vi "Dashboard Main.vi"() -> ()   [LabVIEW 2016]
uses:
  <vilib>/Utility/miscctls.llb/LVRowAndColumnTypeDef.ctl
  <vilib>/event_ctls.llb/eventvkey.ctl
  <vilib>/Rock Robotics/Network Tables/NT Read Boolean.vi
  <vilib>/Rock Robotics/Network Tables/NT Write Boolean.vi
  <vilib>/Rock Robotics/Network Tables/NT Read Numeric Array.vi
  <vilib>/Rock Robotics/WPI/Dashboard/WPI_DashboardLogging Global.vi
panel:
  in  "Camera Settings Right":T1={"Frame Rate"=30, "Compression"=30, "Size"=1, "DB Camera Config"=FALSE} {"Frame Rate" scale=1.0..30.0; "Compression" scale=100.0..-1.0; "Size" items=["640x480", "320x240", "160x120"]}
  in  "Camera Name Right":string(combo)="No Camera Selection"
  out "Camera Info":cluster{"Mbps LED":bool, "Mbps":dbl, "fps":dbl} {"fps" format="%#.1g"; "Mbps" format="%#.1g"}
  in  "Camera Settings":T1={"Frame Rate"=30, "Compression"=30, "Size"=1, "DB Camera Config"=FALSE} {"Frame Rate" scale=1.0..30.0; "Compression" scale=100.0..-1.0; "Size" items=["640x480", "320x240", "160x120"]}
  in  "TCP":refnum<k5>
  in  "Rec Mode":enum32{"Stop", "Record", "Playback"}(radio)
  out "Robot IP":string
  out "Image Message":string="Timeout in Camera Communications"
  in  "Dashboard Tab":T2(tab)
  in  "Select Auto":string(combo)="Select Autonomous ..."
  out "NT Connection":bool
  out "MotorChart R":cluster{"Numeric":dbl, "Numeric":dbl}(graph)
  out "MotorChart L":cluster{"Numeric":dbl, "Numeric":dbl}(graph)
  out "MotorSliders R":cluster{"MotorSlide1":dbl, "MotorSlide2":dbl} {"MotorSlide2" scale=-1.0..1.0 scale format="%#_2e"; "MotorSlide1" scale=-1.0..1.0 scale format="%#_2e"}
  out "MotorSliders L":cluster{"MotorSlide1":dbl, "MotorSlide2":dbl} {"MotorSlide2" scale=-1.0..1.0 scale format="%#_2e"; "MotorSlide1" scale=-1.0..1.0 scale format="%#_2e"}
  out "Gyro":dbl(knob) scale=0.0..360.0
  out "JS1 Z":dbl(slide) scale=-1.0..1.0 scale format="%#_2e"
  out "JS1 Graph":cluster{"X":dbl, "Y":dbl}[](graph)
  out "JS1 Buttons":T3
  out "JS2 Z":dbl(slide) scale=-1.0..1.0 scale format="%#_2e"
  out "JS2 Graph":cluster{"X":dbl, "Y":dbl}[](graph)
  out "JS2 Buttons":T3
  out "Mode":T4(ring)=enum."Auto Disabled"
  out "Camera Image Right":T5(plugin-control)
  in  "DB/String 9":string
  in  "DB/String 8":string
  in  "DB/String 7":string
  in  "DB/String 6":string
  in  "DB/String 5":string
  in  "DB/String 4":string
  in  "DB/String 3":string
  in  "DB/String 2":string
  in  "DB/String 1":string
  in  "DB/String 0":string
  in  "DB/Slider 0":dbl(slide) scale=0.0..5.0
  in  "DB/Slider 1":dbl(slide) scale=0.0..5.0
  in  "DB/Slider 2":dbl(slide) scale=0.0..5.0
  in  "DB/Slider 3":dbl(slide) scale=0.0..5.0
  out "DB/LED 3":bool
  out "DB/LED 2":bool
  out "DB/LED 1":bool
  out "DB/LED 0":bool
  in  "DB/Button 3":bool
  in  "DB/Button 2":bool
  in  "DB/Button 1":bool
  in  "DB/Button 0":bool caption="New Name"
  in  "Capture":bool=TRUE
  in  "Test Slider":dbl(slide) scale=0.0..100.0 scale format="%#_3g"
  in  "On/Off":bool caption="Solenoid"
  in  "Test Name":u16(ring) items=["Select the test to run..."]
  in  "Test Tree":string(tree)
  in  "Motor":cluster{"Value":dbl, "Enable":bool} {"Value" scale=-1.0..1.0 scale format="%#_3g"}
  out "Progress":T6 {"Test Progress" scale=0.0..100.0}
  in  "Rev/Fwd":cluster{"Forward":bool, "Reverse":bool}
  in  "Test Ring":u16(ring) items=["Monochrome", "Color"]
  out "Cmd Status":string
  in  "Execute Command":bool
  in  "Command Params":string[][](table)
  in  "Command Selection":i32(listbox)
  in  "CheckList":i32(listbox)
  out "Tree":string(tree)
  out "Camera Image":T5(plugin-control)
  out "Background":bool
  in  "Camera Name":string(combo)="No Camera Selection"
  # "HW"
  # "HW"
  # "Joysticks"
  # "Drive Motors"
  # "Front"
  # "Right"
  # "Left"
  # "Back"
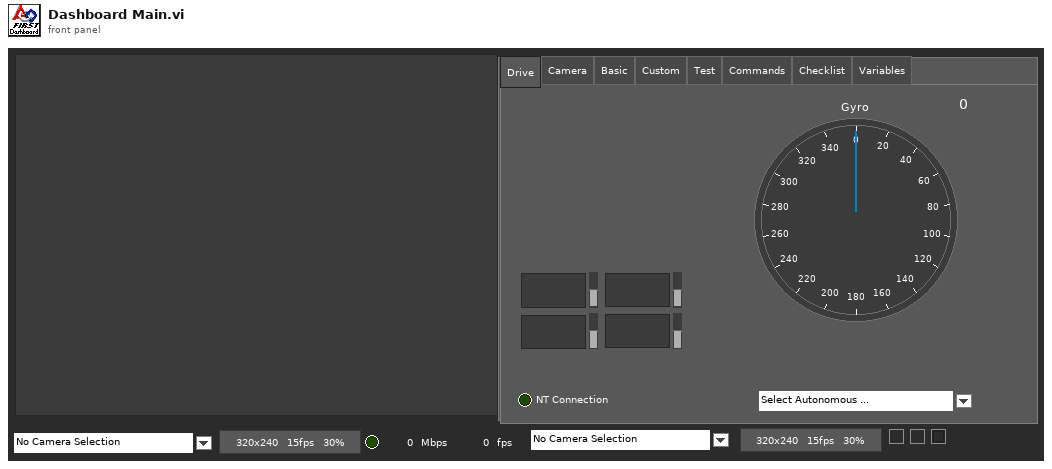
[diagram p1: front panel]
types:
  T1 = cluster{"Frame Rate":i32, "Compression":i32, "Size":u16, "DB Camera Config":bool}
  T2 = enum32{"Drive", "Camera", "Basic", "Custom", "Test", "Commands", "Checklist", "Variables"}
  T3 = cluster{bool, bool, bool, bool, bool, bool, bool, bool, bool, bool, bool, bool}
  T4 = enum8{"Tele-Op Disabled", "Tele-Op Enabled", "Auto Disabled", "Auto Enabled", "Test Disabled", "Test Enabled", "Disconnected", "No Code", "E-Stop"}
  T5 = typedef "IMAQ Image.ctl" = refnum<image>
  T6 = cluster{"Test Progress":u8, "Test Progress Text":string}
  T7 = typedef "Image Type" = u32
  T8 = cluster{"IDs":cluster{"RPC field ID":u16, "Unique ID":u16}, "String":string}
  T9 = enum32{"Drive", "Basic", "Custom", "Test", "Checklist", "Variables"}
  T10 = enum16{"open", "replace", "create", "open or create", "replace or create", "replace or create with confirmation"}
  T11 = cluster{"Error Strings":string, "Disable Counts":cluster{u16, u16}, "Rail Faults":cluster{u16, u16, u16}, "Robot IP":string, "DB Mode":u8, "Event Info":cluster{"Name":string, "Type":u8, "Number":u16, "Replay":u8}}
  T12 = cluster{"Storage":cluster{"Disk Free":u64, "RAM Block":u32, "RAM free":u32}, "CPU Utilization":cluster{"CPU % ISR":sgl, "CPU % Time Crit":sgl, "CPU % Timed Str":sgl, "CPU % High":sgl, "CPU % Above":sgl, "CPU % Normal":sgl, "CPU % Low":sgl}, "CAN":cluster{"% Bus Utilization":sgl, "Bus Off Cnt":u32, "TX_FIFO Full Cnt":u32, "Receive Error Cnt":u8, "Transmit Error Cnt":u8}, "HID":cluster{"HID Outputs":u32, "Rumble Low":u16, "Rumble High":u16}[]}
  T13 = cluster{"Status bits":cluster{"Test Mode":bool, "Autonomous":bool, "Enabled":bool, "Code Start":bool, "Brownout":bool, "Reserved 2":bool, "Reserved 3":bool, "E-Stop":bool}, "Code Trace":cluster{"Disabled":bool, "TeleOp":bool, "Auto":bool, "Test":bool}, "Controller Type":enum16{"unknown", "cRIO", "roboRio"}, "Code?":enum16{"unknown", "noCode", "code"}, "Battery V":dbl}
  T14 = cluster{"Control Bits":cluster{"TestMode":bool, "Autonomous":bool, "Enabled":bool, "FMS Present":bool, bool, bool, bool, "E-Stop":bool}, "Team Station ":u8, "Countdown":sgl, "Joystick Values":cluster{"Axes":dbl[], "Buttons":bool[], "POVs":i16[]}[]}
  T15 = cluster{"Axes":dbl[], "Buttons":bool[], "POVs":i16[]}[]
  T16 = cluster{"Axes":dbl[], "Buttons":bool[], "POVs":i16[]}
  T17 = cluster{"Buttons[0]":bool, "Buttons[1]":bool, "Buttons[2]":bool, "Buttons[3]":bool, "Buttons[4]":bool, "Buttons[5]":bool, "Buttons[6]":bool, "Buttons[7]":bool, "Buttons[8]":bool, "Buttons[9]":bool, "Buttons[10]":bool, "Buttons[11]":bool}
  T18 = cluster{"Camera Image":refnum<vi>, "Dashboard Tab":refnum<vi>, "Background":refnum<vi>, "Rec Mode":refnum<vi>, "Test Slider":refnum<vi>, "On/Off ":refnum<vi>, "Test Ring":refnum<vi>, "Rev/Fwd":refnum<vi>, "Test Name":refnum<vi>, "Motor":refnum<vi>, "Progress":refnum<vi>, "CheckList":refnum<vi>, "Tree":refnum<vi>, "Test Tree":refnum<vi>, "Command Params":refnum<vi>, "Command Selection":refnum<vi>, "Execute Command":refnum<vi>, "Cmd Status":refnum<vi>, "Camera Settings":refnum<vi>, "Camera Name":refnum<vi>, "Camera Info":refnum<vi>, "Camera Settings Right":refnum<vi>, "Camera Name Right":refnum<vi>, "Camera Image Right":refnum<vi>}
  T19 = cluster{"Operation":enum16{"Update", "Clear"}, "Color Box":u32}[]
  T20 = typedef "eventvkey.ctl" = enum16{"ASCII", "Enter", "Return", "Shift", "Ctrl", "Alt", "Cmd", "Opt", "Caps", "NumLock", "Clear", "Break", "Up", "Down", "Left", "Right", "Insert", "Delete", "Home", "End", "PageUp", "PageDown", "Escape", "Help", "Pause", "ScrollLock", "F1", "F2", "F3", "F4", "F5", "F6", "F7", "F8", "F9", "F10", "F11", "F12", "F13", "F14", "F15", "F16", "F17", "F18", "F19", "F20", "F21", "F22", "F23", "F24", "Play", "VolumeUp", "VolumeDown", "Mute", "Two Byte Char"}
  T21 = cluster{"Image Size":bool, "Image Type":bool, "Pixel Value":bool, "ROI Information":bool, "Zoom Factor":bool}
  T22 = cluster{"Operation":enum16{"Update", "Clear"}, "Color Box":u32}
  T23 = typedef "LVRowAndColumnTypeDef.ctl" = cluster{"Row":i32, "Column":i32}
  T24 = cluster{"Shift":bool, "Ctrl":bool, "Alt":bool, "Cmd":bool, "Opt":bool}
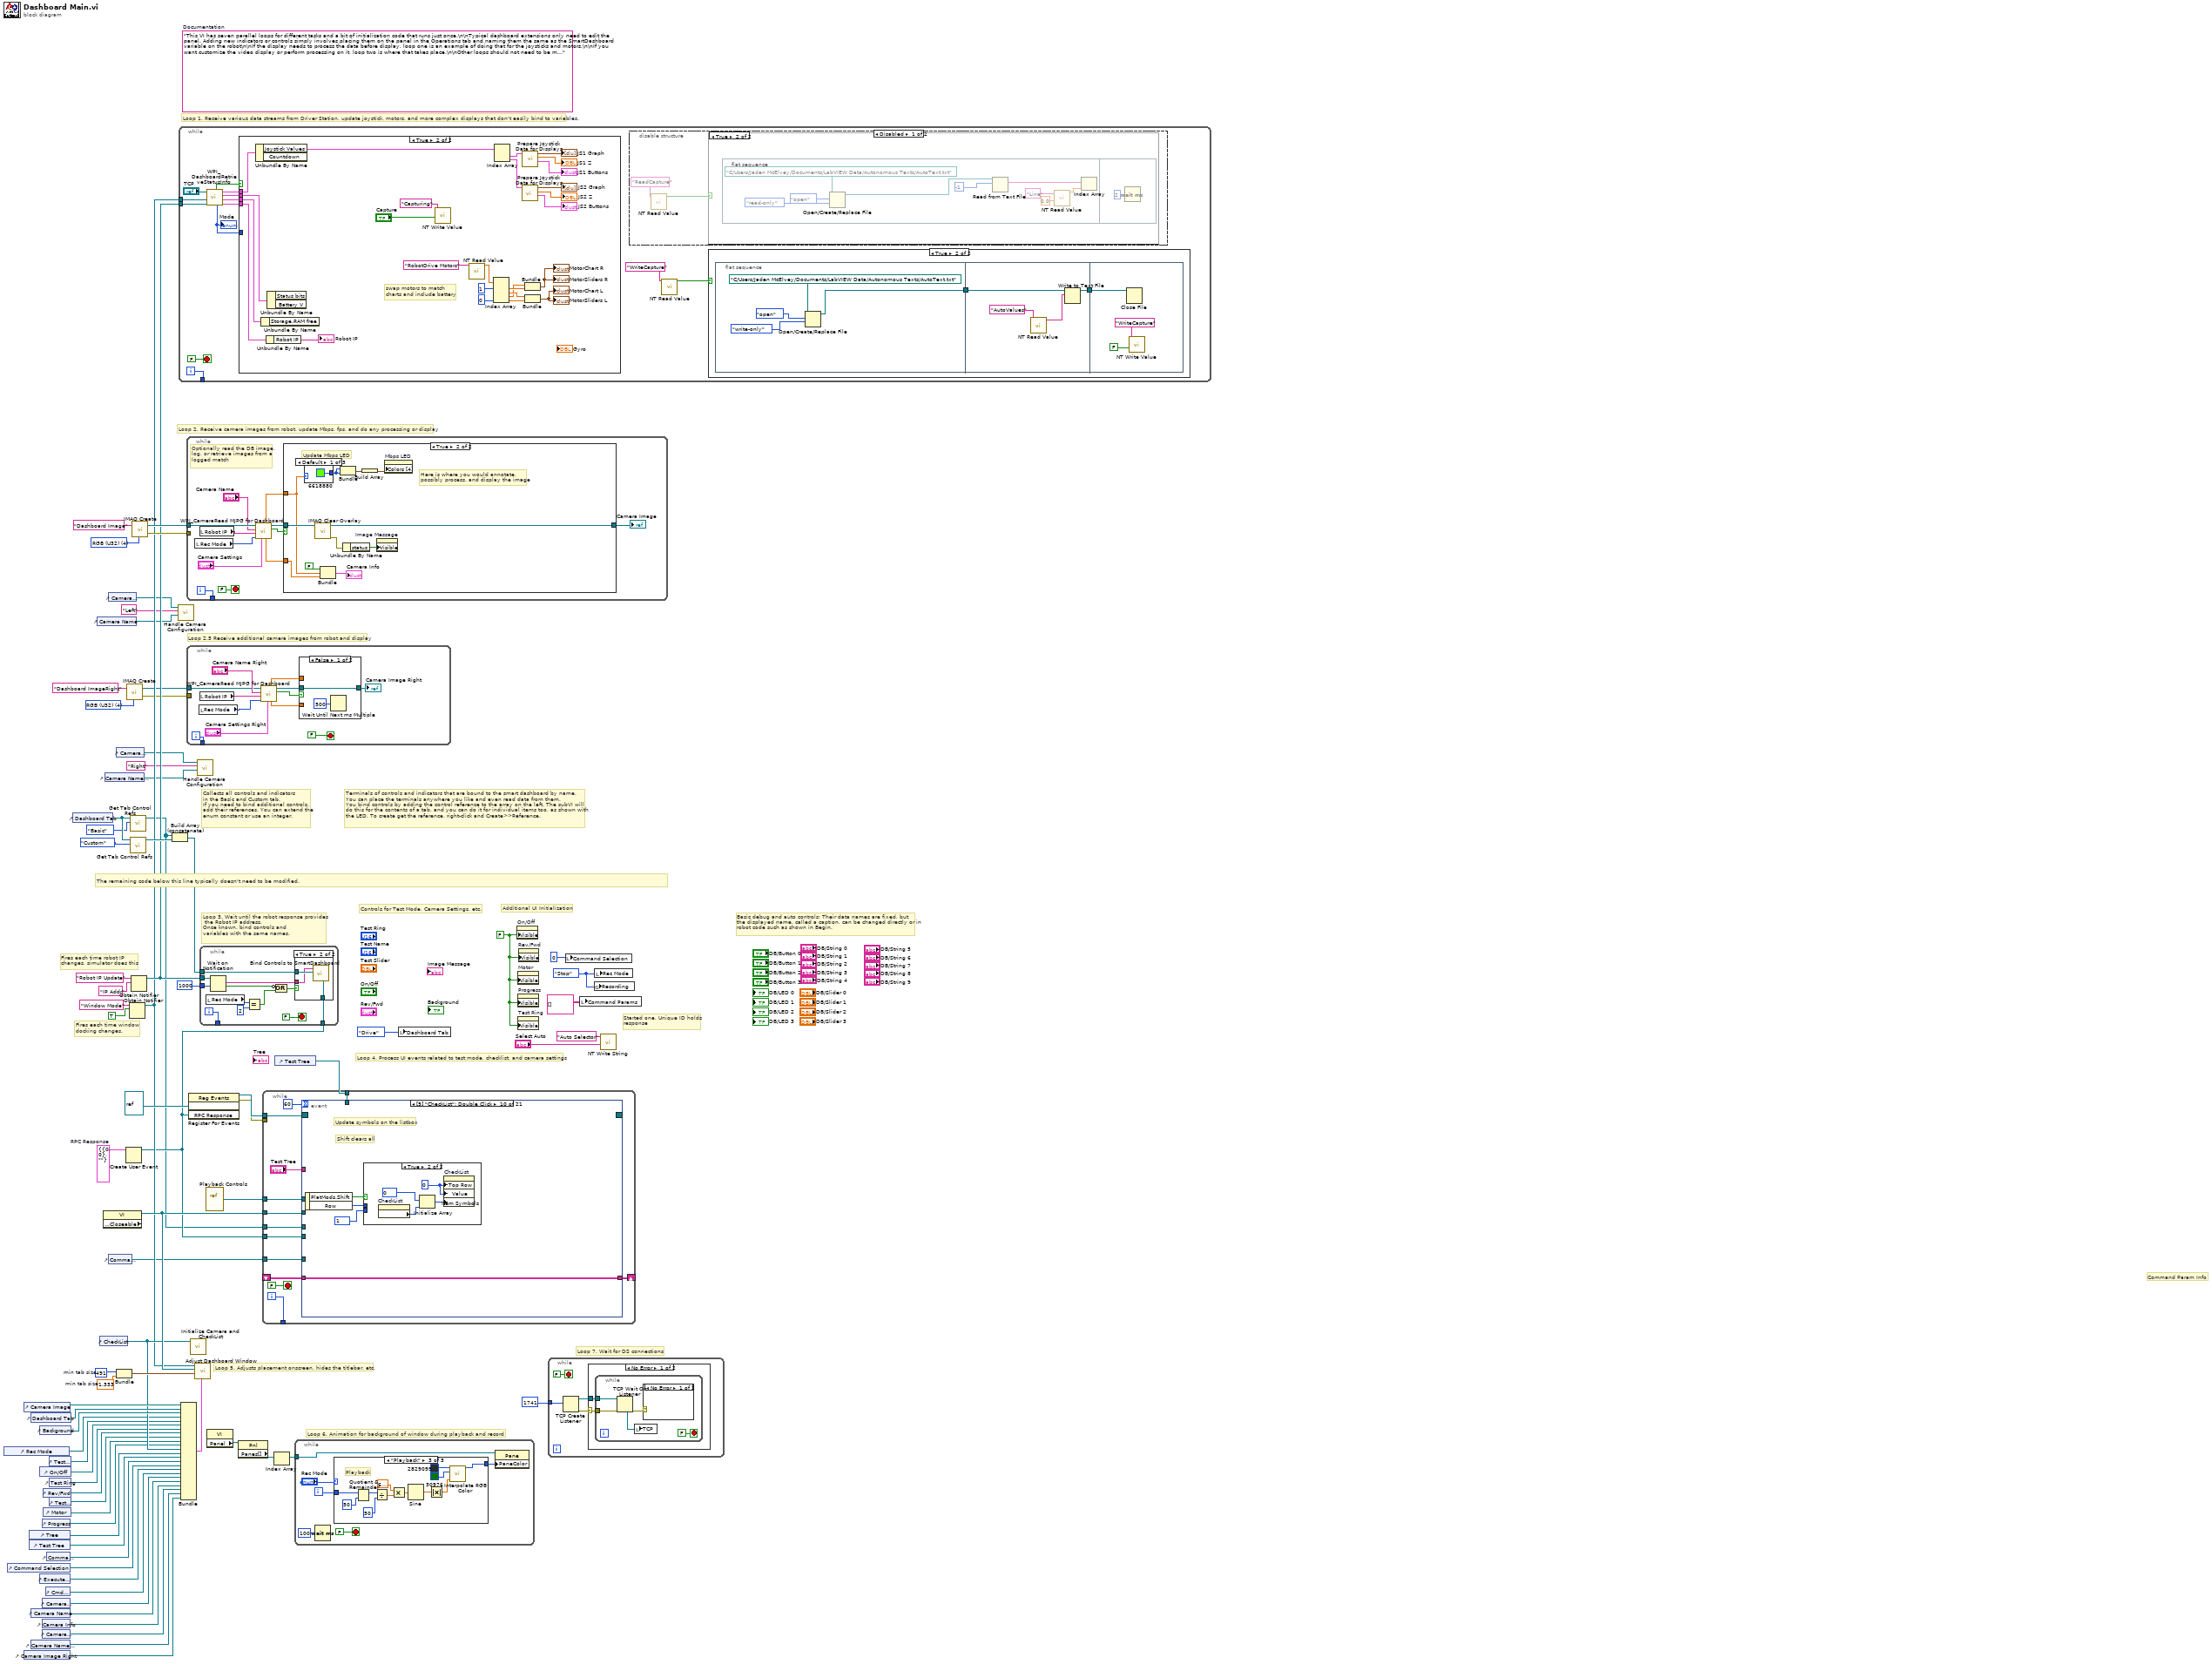
[diagram p0: block diagram]
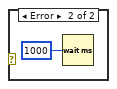
[diagram p3: hidden frame]
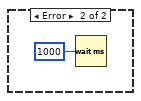
[diagram p4: hidden frame]
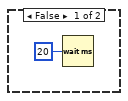
[diagram p8: hidden frame]
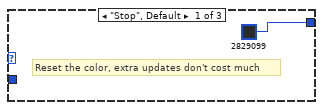
[diagram p9: hidden frame]
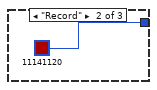
[diagram p10: hidden frame]
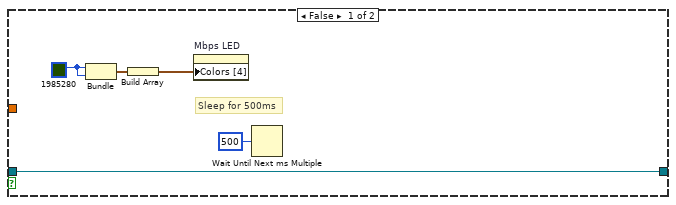
[diagram p12: hidden frame]
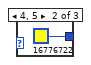
[diagram p13: hidden frame]
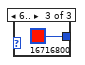
[diagram p14: hidden frame]
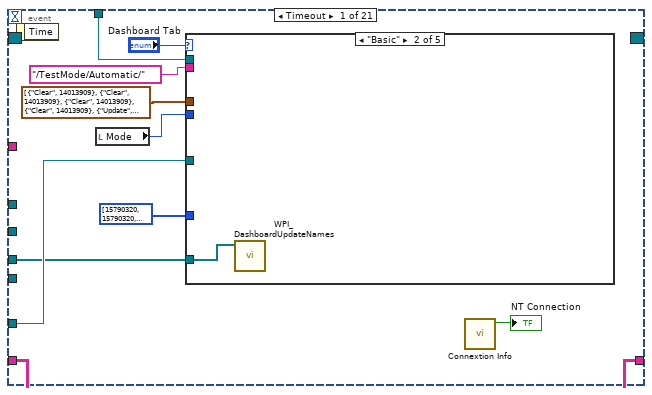
[diagram p15: hidden frame]
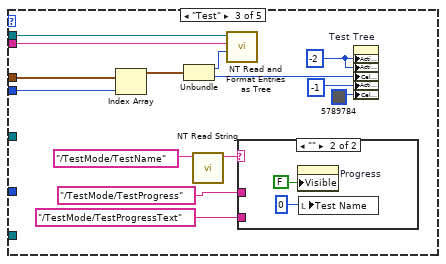
[diagram p17: hidden frame]
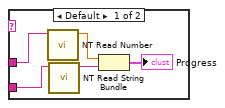
[diagram p18: hidden frame]
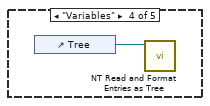
[diagram p19: hidden frame]
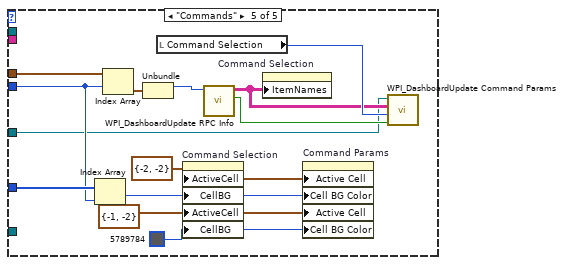
[diagram p20: hidden frame]
diagram:
  w11 = T7 4 items=["Grayscale (U8)", "Grayscale (I16)", "Grayscale (SGL)", "Complex (CSG)", "RGB (U32)", "HSL (U32)", "RGB (U64)"] ("Image Type")
  w26 = T8 {"IDs"={"RPC field ID"=0, "Unique ID"=0}, "String"=""}  # RPC Response
  w51 = 491  # min tab size
  w50 = 1.333  # min tab size
  w58 = enum32{"Stop", "Record", "Playback"}."Stop" ("Rec Mode")
  w33 = FALSE ("Visible")
  (unwired) "This VI has seven parallel loops for different tasks and a bit of initialization code that runs just once.\n\nTypical dashboard extensions only need to edit the panel. Adding new indicators or controls simply involves placing them on the panel in the Operations tab and naming them the same as the SmartDashboard variable on the robot\n\nIf the display needs to process the data before display, loop one is an example of doing that for the joysticks and motors.\n\nIf you want customize the video display or perform processing on it, loop two is where that takes place.\n\nOther loops should not need to be modified. They are pretty standard, and document the task they perform."  # Documentation
  w75 = T7 4 items=["Grayscale (U8)", "Grayscale (I16)", "Grayscale (SGL)", "Complex (CSG)", "RGB (U32)", "HSL (U32)", "RGB (U64)"] ("Image Type")
  # "Loop 2.5 Receive additional camera images from robot and display"
  # "Command Param Info"
  # "Started one, Unique ID holds\nresponse"
  # "Loop 7. Wait for DS connections"
  # "Basic debug and auto controls: Their data names are fixed, but\nthe displayed name, called a caption, can be changed directly or in\nrobot code such as shown in Begin."
  # "Controls for Test Mode, Camera Settings, etc."
  # "Additional UI Initialization"
  # "Loop 6. Animation for background of window during playback and record"
  # "Fires each time robot IP\nchanges, simulator does this"
  # "Fires each time window\ndocking changes."
  # "Collects all controls and indicators\nin the Basic and Custom tab.\nIf you need to bind additional controls,\nadd their references. You can extend the\nenum constant or use an integer."
  # "The remaining code below this line typically doesn't need to be modified."
  # "Loop 4. Process UI events related to test mode, checklist, and camera settings"
  # "Terminals of controls and indicators that are bound to the smart dashboard by name.\nYou can place the terminals anywhere you like and even read data from them.\nYou bind controls by adding the control reference to the array on the left. The subVI will\ndo this for the contents of a tab, and you can do it for individual items too, as shown with\nthe LED. To create get the reference, right-click and Create>>Reference."
  # "Loop 3. Wait until the robot response provides\n the Robot IP address.\nOnce known, bind controls and\nvariables with the same names."
  # "Loop 5. Adjusts placement onscreen, hides the titlebar, etc."
  # "Loop 1. Receive various data streams from Driver Station, update joystick, motors, and more complex displays that don't easily bind to variables."
  # "Loop 2. Receive camera images from robot, update Mbps, fps, and do any processing or display"
  n1 = control-ref of="Rec Mode"() -> (w39:refnum<vi>)
  n2 = control-ref of="Command Selection"() -> (w25:refnum<vi>)
  n3 = control-ref of="Camera Image Right"() -> (w2:refnum<vi>)
  n4 = control-ref of="Camera Image"() -> (w53:refnum<vi>)
  n5 = control-ref of="Tree"() -> (w43:refnum<vi>)
  n6 = control-ref of="Test Tree"() -> (w42:refnum<vi>)
  n7 = control-ref of="Dashboard Tab"() -> (w52:refnum<vi>)
  n8 = control-ref of="Camera Name"() -> (w16:refnum<vi>)
  n9 = control-ref of="Camera Name Right"() -> (w3:refnum<vi>)
  n10 = control-ref of="Execute Command"() -> (w27:refnum<vi>)
  n11 = control-ref of="Background"() -> (w48:refnum<vi>)
  n12 = control-ref of="On/Off"() -> (w37:refnum<vi>)
  n13 = control-ref of="Progress"() -> (w34:refnum<vi>)
  n14 = control-ref of="Camera Settings"() -> (w17:refnum<vi>)
  n15 = control-ref of="Camera Info"() -> (w15:refnum<vi>)
  n16 = control-ref of="Camera Settings Right"() -> (w4:refnum<vi>)
  n17 = control-ref of="Rev/Fwd"() -> (w35:refnum<vi>)
  n18 = control-ref of="Motor"() -> (w40:refnum<vi>)
  n19 = control-ref of="Cmd Status"() -> (w21:refnum<vi>)
  n20 = control-ref of="Command Params"() -> (w28:refnum<vi>)
  n21 = control-ref of="Test Slider"() -> (w38:refnum<vi>)
  n22 = control-ref of="Test Ring"() -> (w36:refnum<vi>)
  n23 = control-ref of="Test Name"() -> (w41:refnum<vi>)
  n24 = control-ref of="Dashboard Tab"() -> (w56:refnum<vi>)
  n25 = control-ref of="Camera Name"() -> (w18:refnum<vi>)
  n26 = control-ref of="CheckList"() -> (w44:refnum<vi>)
  n27 = property class="VI" props=["Front Panel.Closeable"]() -> (reference out=w57:refnum<vi>)  [unwired: 2 in, 2 out]
  n28 = control-ref of="Camera Name Right"() -> (w7:refnum<vi>)
  n29 = control-ref of="Camera Settings"() -> (w19:refnum<vi>)
  n30 = control-ref of="Command Params"() -> (w20:refnum<vi>)
  n31 = control-ref of="Camera Settings Right"() -> (w8:refnum<vi>)
  n32 = Bundle("min tab size"=w51, "min tab size"=w50) -> (w49:cluster{"min tab size":i32, "min tab size":dbl})  [unwired: 1 in]
  n33 = Create User Event(user event datatype=w26) -> (user event=w22:refnum<user-event>)  [unwired: 1 in, 1 out]
  n34 = call "IMAQ Create"("Image Name"="Dashboard ImageRight", "Image Type"=w11) -> ("New Image"=w10:T5, "error out"=w9:errorcluster)  [unwired: 2 in, 1 out]
  n35 = Obtain Notifier(name (unnamed)="Window Mode", notification data type=TRUE) -> (notifier out=w31:refnum<notifier>)  [unwired: 2 in, 2 out]
  n36 = call <vilib>:"Get Tab Control Refs.vi"("Page Index"=T9."Basic" ("Dashboard Tab"), "TabControl in"=w56) -> ("ControlsOnPage"=w14:refnum<vi>[])  [unwired: 9 in]
  n37 = call <vilib>:"Get Tab Control Refs.vi"("Page Index"=T9."Custom" ("Dashboard Tab"), "TabControl in"=w56) -> ("ControlsOnPage"=w55:refnum<vi>[])  [unwired: 9 in]
  n38 = Obtain Notifier(name (unnamed)="Robot IP Update", notification data type="IP Addr" ("name (unnamed)")) -> (notifier out=w32:refnum<notifier>)  [unwired: 2 in, 2 out]
  n39 = call "IMAQ Create"("Image Name"="Dashboard Image", "Image Type"=w75) -> ("New Image"=w73:T5, "error out"=w72:errorcluster)  [unwired: 2 in, 1 out]
  n40 = Build Array (concatenate)(w14, w55) -> (w54:refnum<vi>[])
  n41 = call "Handle Camera Configuration.vi"("CameraNameRef"=w18, "Camera File Name"="Left", "ClusterRef"=w19) -> ()  [unwired: 9 in]
  n42 = while {
    tunnel: [w87] -> _
    tunnel: w32 -> [w81]
    tunnel: w31 -> [w78]
    i -> [w87]
    stop <- FALSE stop-if-true
    n43 = call <vilib>:"WPI_DashboardRetrieveStatusInfo.vi"("Binding Refnum"=w81, "Window Mode Notifier"=w78, "TCP Cnx"="TCP") -> ("Power and Errors"=w82:T11, "Robot Metrics"=w85:T12, "Status Info"=w86:T13, "Control Info"=w83:T14, "Robot Mode"=w80:T4, "Process?"=w84:bool)  [unwired: 3 in]
    "Mode" <- w80
    n44 = case shown="True" w84 {
      tunnel: w86 -> [_ w140]
      tunnel: w85 -> [_ w139]
      tunnel: w83 -> [_ w138]
      tunnel: w82 -> [_ w137]
      tunnel: w80 -> [_ _]
      frame False {
        n45 = Wait (ms)(milliseconds to wait=u32 20) -> ()  [unwired: 1 out]
      }
      frame True {
        # "swap motors to match\ncharts and include battery"
        n46 = Unbundle By Name(w138) -> ("Joystick Values"=w128:T15)  [unwired: 1 out]
        n47 = Unbundle By Name(w139) -> ()  [unwired: 1 out]
        n48 = Unbundle By Name(w137) -> ("Robot IP"=→"Robot IP":string)
        n49 = Unbundle By Name(w140) -> ()  [unwired: 2 out]
        n50 = call-poly <vilib>:"NT Write Value.vi"("Boolean"="Capture", "Name"="Capturing") -> ()  [unwired: 9 in, 1 out]
        n51 = call-poly <vilib>:"NT Read Value.vi"("Name"="RobotDrive Motors") -> ("Numeric Array"=w118:dbl[])  [unwired: 9 in, 1 out]
        n52 = Index Array(array=w118, index #1=1, index #4=0) -> (element #1=w132:dbl, element #2=w133:dbl, element #3=w131:dbl, element #4=w136:dbl)  [unwired: 2 in]
        n53 = Index Array(array=w128) -> (element #1=w127:T16, element #2=w123:T16)  [unwired: 2 in]
        n54 = call "Prepare Joystick Data for Displays.vi"("Joystick Values"=w123) -> ("Buttons"=→"JS2 Buttons":T17, "Z Axis"=→"JS2 Z":dbl, "Cartesian Data"=→"JS2 Graph":cluster{"X axis":dbl, "X axis":dbl}[])  [unwired: 8 in]
        n55 = call "Prepare Joystick Data for Displays.vi"("Joystick Values"=w127) -> ("Buttons"=→"JS1 Buttons":T17, "Z Axis"=→"JS1 Z":dbl, "Cartesian Data"=→"JS1 Graph":cluster{"X axis":dbl, "X axis":dbl}[])  [unwired: 8 in]
        n56 = Bundle("Numeric"=w131, "Numeric"=w132) -> (→"MotorChart R" →"MotorSliders R":cluster{"Numeric":dbl, "Numeric":dbl})  [unwired: 1 in]
        n57 = Bundle("Numeric"=w133, "Numeric"=w136) -> (→"MotorChart L" →"MotorSliders L":cluster{"Numeric":dbl, "Numeric":dbl})  [unwired: 1 in]
      }
    }
    n58 = disable-structure shown="Disabled" {
      frame Disabled {
        n59 = call-poly <vilib>:"NT Read Value.vi"("Name"="ReadCapture") -> ("Boolean"=w89:bool)  [unwired: 9 in, 1 out]
        n60 = case shown="True" w89 {
          frame False {
          }
          frame True {
            n61 = flat-sequence {
              frame #0 {
                n62 = Open/Create/Replace File(file path (use dialog)=path "C:/Users/Jaden McElvey/Documents/LabVIEW Data/Autonomous Texts/AutoText.txt", operation (0:open)=T10."open", access (0:read/write)=enum16{"read/write", "read-only", "write-only"}."read-only") -> (refnum out=w91:refnum<file>)  [unwired: 3 in, 2 out]
                n63 = Read from Text File(file (use dialog)=w91, count=-1) -> (text=w98:string[])  [unwired: 2 in, 3 out]
                n64 = call-poly <vilib>:"NT Read Value.vi"("Default Value"=0.0, "Name"="Line") -> ("Numeric"=w95:dbl)  [unwired: 8 in, 1 out]
                n65 = Index Array(array=w98, index=w95) -> ()  [unwired: 1 out]
              }
              frame #1 {
                n66 = Wait (ms)(milliseconds to wait=u32 2) -> ()  [unwired: 1 out]
              }
            }
          }
        }
      }
      frame Enabled {
      }
    }
    n67 = call-poly <vilib>:"NT Read Value.vi"("Name"="WriteCapture") -> ("Boolean"=w77:bool)  [unwired: 9 in, 1 out]
    n68 = case shown="True" w77 {
      frame False {
      }
      frame True {
        n69 = flat-sequence {
          tunnel: [w103] -> w102
          tunnel: w102 -> [w108]
          tunnel: [w109] -> w101
          tunnel: w101 -> [w113]
          frame #0 {
            n70 = Open/Create/Replace File(file path (use dialog)=path "C:/Users/Jaden McElvey/Documents/LabVIEW Data/Autonomous Texts/AutoText.txt", operation (0:open)=T10."open", access (0:read/write)=enum16{"read/write", "read-only", "write-only"}."write-only") -> (refnum out=w103:refnum<file>)  [unwired: 3 in, 2 out]
          }
          frame #1 {
            n71 = call-poly <vilib>:"NT Read Value.vi"("Name"="AutoValues") -> ("String"=w107:string)  [unwired: 9 in, 1 out]
            n72 = Write to Text File(file (use dialog)=w108, text=w107) -> (refnum out=w109:refnum<file>)  [unwired: 2 in, 2 out]
          }
          frame #2 {
            n73 = Close File(refnum=w113) -> ()  [unwired: 1 in, 2 out]
            n74 = call-poly <vilib>:"NT Write Value.vi"("Boolean"=FALSE, "Name"="WriteCapture") -> ()  [unwired: 9 in, 1 out]
          }
        }
      }
    }
  }
  n75 = Bundle("Camera Image"=w53, "Dashboard Tab"=w52, "Background"=w48, "Rec Mode"=w39, "Test Slider"=w38, "On/Off"=w37, "Test Ring"=w36, "Rev/Fwd"=w35, "Test Name"=w41, "Motor"=w40, "Progress"=w34, "CheckList"=w44, "Tree"=w43, "Test Tree"=w42, "Command Params"=w28, "Command Selection"=w25, "Execute Command"=w27, "Cmd Status"=w21, "Camera Settings"=w17, "Camera Name"=w16, "Camera Info"=w15, "Camera Settings Right"=w4, "Camera Name Right"=w3, "Camera Image Right"=w2) -> (w45:T18)  [unwired: 1 in]
  n76 = while {
    tunnel: w73 -> [w150]
    tunnel: w72 -> [_]
    tunnel: [w151] -> _
    i -> [w151]
    stop <- FALSE stop-if-true
    # "Optionally read the DB image,\nlog, or retrieve images from a\nlogged match"
    n77 = local read "Rec Mode"() -> (w146:enum32{"Stop", "Record", "Playback"})
    n78 = local read "Robot IP"() -> (w145:string)
    n79 = call <vilib>:"WPI_CameraRead MJPG for Dashboard.vi"("Camera Settings"="Camera Settings", "Rec Mode"=w146, "Robot IP"=w145, "Camera Name"="Camera Name", "Refnum in"=w150) -> ("Active"=w148:bool, "Refnum out"=w149:T5, "FPS"=w147:dbl, "Bandwidth (Mbps)"=w144:dbl)  [unwired: 3 in]
    n80 = case shown="True" w148 {
      tunnel: w149 -> [w153 w164]
      tunnel: w144 -> [_ w161]
      tunnel: w147 -> [_ w162]
      tunnel: [w153 w158] -> w141
      frame False {
        w155 = u32 1985280 ("Color Box")
        # "Sleep for 500ms"
        n81 = Bundle("Color Box"=w155, "Color Box"=w155) -> (w156:cluster{"Color Box":u32, "Color Box":u32})  [unwired: 1 out]
        n82 = Build Array(w156) -> (w154:cluster{"Color Box":u32, "Color Box":u32}[])
        n83 = property on="Mbps LED" class="Bool (strict)"("Colors [4]"=w154) -> ()  [unwired: 2 in, 2 out]
        n84 = Wait Until Next ms Multiple(millisecond multiple=u32 500) -> ()  [unwired: 1 out]
      }
      frame True {
        # "Here is where you would annotate,\npossibly process, and display the image"
        # "Update Mbps LED"
        n85 = case shown="Default" w161 {
          tunnel: [u32 6618880 ("Color Box") u32 16776722 ("Color Box") u32 16716800 ("Color Box")] -> w165
          frame Default {
          }
          frame 4, 5 {
          }
          frame 6.. {
          }
        }
        n86 = call "IMAQ Clear Overlay"("Image"=w164) -> ("error out"=w167:errorcluster, "Image Out"=w158:T5)  [unwired: 2 in, 7 out]
        n87 = Bundle(FALSE, "Bandwidth (Mbps)"=w161, "FPS"=w162) -> (→"Camera Info":cluster{bool, "Bandwidth (Mbps)":dbl, "FPS":dbl})  [unwired: 1 in]
        n88 = Bundle("Color Box"=w165, "Color Box"=w165) -> (w166:cluster{"Color Box":u32, "Color Box":u32})  [unwired: 1 out]
        n89 = Unbundle By Name(w167) -> ("status"=w168:bool)
        n90 = Build Array(w166) -> (w163:cluster{"Color Box":u32, "Color Box":u32}[])
        n91 = property on="Image Message" class="Str"("Visible"=w168) -> ()  [unwired: 2 in, 2 out]
        n92 = property on="Mbps LED" class="Bool (strict)"("Colors [4]"=w163) -> ()  [unwired: 2 in, 2 out]
      }
    }
    "Camera Image" <- w141
  }
  n93 = while {
    tunnel: w10 -> [w182]
    tunnel: w9 -> [_]
    tunnel: [w176] -> _
    i -> [w176]
    stop <- FALSE stop-if-true
    n94 = local read "Rec Mode"() -> (w180:enum32{"Stop", "Record", "Playback"})
    n95 = local read "Robot IP"() -> (w181:string)
    n96 = call <vilib>:"WPI_CameraRead MJPG for Dashboard.vi"("Camera Settings"="Camera Settings Right", "Rec Mode"=w180, "Robot IP"=w181, "Camera Name"="Camera Name Right", "Refnum in"=w182) -> ("Active"=w175:bool, "Refnum out"=w178:T5, "FPS"=w173:dbl, "Bandwidth (Mbps)"=w174:dbl)  [unwired: 3 in]
    n97 = case shown="False" w175 {
      tunnel: w178 -> [w184 w186]
      tunnel: w174 -> [_ _]
      tunnel: w173 -> [_ _]
      tunnel: [w184 w186] -> w172
      frame False {
        n98 = Wait Until Next ms Multiple(millisecond multiple=u32 500) -> ()  [unwired: 1 out]
      }
      frame True {
      }
    }
    "Camera Image Right" <- w172
  }
  n99 = register-events(refnum<vi> refnum, w22) -> (reference out=w62:refnum<event-registration>, error out=w61:errorcluster)  [unwired: 2 in]
  n100 = call "Initialize Camera and CheckList.vi"("ListBox in"=w44) -> ()  [unwired: 11 in]
  n101 = call "Adjust Dashboard Window.vi"("Sizing Refnums"=w45, "Size Constraints"=w49, "VI"=w57, "WIn Mode"=w31) -> ()  [unwired: 8 in]
  n102 = call "Handle Camera Configuration.vi"("CameraNameRef"=w7, "Camera File Name"="Right", "ClusterRef"=w8) -> ()  [unwired: 9 in]
  n103 = while {
    tunnel: w54 -> [w198]
    tunnel: w32 -> [w196]
    tunnel: [w194] -> _
    tunnel: u32 1000 ("milliseconds to wait") -> [w193]
    tunnel: w22 -> [w187]
    i -> [w194]
    stop <- FALSE stop-if-true
    n104 = local read "Rec Mode"() -> (w189:enum32{"Stop", "Record", "Playback"})
    n105 = Wait on Notification(notifier=w196, timeout in ms (-1)=w193) -> (notification=w195:string, timed out?=w191:bool)  [unwired: 2 in, 2 out]
    n106 = Equal?(x=w189, y=u16 2 ("Rec Mode")) -> (x = y?=w190:bool)
    n107 = Compound Arithmetic op=OR(invert w191, w190) -> (w192:bool)
    n108 = case shown="True" w192 {
      tunnel: w198 -> [_ w201]
      tunnel: w195 -> [_ w200]
      tunnel: w187 -> [_ w199]
      frame False {
      }
      frame True {
        n109 = call <vilib>:"Bind Controls to SmartDashboard.vi"("RPC ref"=w199, "Bound Control Refs"=w201, "Server IP Address"=w200) -> ()  [unwired: 9 in]
      }
    }
  }
  n110 = vi-ref "Playback Controls.vi"() -> (w63:refnum<vi>)
  n111 = property class="VI"() -> ("Panel"=w65:refnum<vi>)  [unwired: 2 in, 2 out]
  n112 = property class="Pnl"(reference=w65) -> ("Panes[]"=w66:refnum<vi>[])  [unwired: 1 in, 2 out]
  n113 = Index Array(array=w66) -> (element=w64:refnum<vi>)  [unwired: 1 in]
  n114 = control-ref of="Test Tree"() -> (w67:refnum<vi>)
  n115 = while {
    tunnel: [w211] -> _
    tunnel: w67 -> [w210]
    tunnel: w63 -> [w209]
    tunnel: w62 -> [w208]
    tunnel: w61 -> [_]
    tunnel: w57 -> [w207]
    tunnel: w22 -> [w206]
    tunnel: w20 -> [w205]
    shift-right: [w204] -> _
    shift-left: _ -> [w203]
    tunnel: w14 -> [w202]
    i -> [w211]
    stop <- FALSE stop-if-true
    n116 = event shown="[9] \"CheckList\": Double Click" {
      selector: w208 -> [_ _ _ _ _ _ _ _ _ _ _ _ _ _ _ _ _ _ _ _ _]
      dyn-events: [_ _ _ _ _ _ _ _ _ _ _ _ _ _ _ _ w467 _ _ _ _] -> _
      timeout: u32 60 ("milliseconds to wait") -> [_ _ _ _ _ _ _ _ _ _ _ _ _ _ _ _ _ _ _ _ _]
      tunnel: w210 -> [w223 _ _ _ _ _ _ _ _ _ _ _ _ _ _ _ _ _ _ _ _]
      tunnel: "Test Tree" -> [_ _ _ _ _ _ _ _ _ _ _ w434 w442 w444 w448 w456 _ _ _ _ _]
      tunnel: w209 -> [_ _ _ _ _ _ _ _ _ _ _ _ _ _ _ _ w469 _ w487 _ _]
      tunnel: w207 -> [_ _ _ _ _ _ _ _ _ _ _ _ _ _ _ _ w465 _ _ _ _]
      tunnel: w206 -> [_ _ _ _ _ _ _ _ _ _ _ _ _ _ _ _ w461 _ _ _ _]
      tunnel: w205 -> [w218 _ _ _ _ _ w385 _ _ _ _ _ _ _ _ _ _ _ _ _ _]
      tunnel: [w217 w262 w364 w369 w378 w382 w383 w392 w402 w409 w421 w433 w440 w443 w447 w455 w460 w482 w484 w488 w499] -> w204
      tunnel: w203 -> [w217 w262 w364 w369 w378 w382 w383 _ _ w409 w421 w433 w440 w443 w447 w455 w460 w482 w484 w488 w499]
      tunnel: w202 -> [w215 _ _ _ _ _ _ _ _ _ _ _ _ _ _ _ _ _ _ _ _]
      event Timeout {
        n117 = event-data() -> ()  [unwired: 1 in, 1 out]
        n118 = local read "Mode"() -> (w220:T4)
        n119 = case shown="\"Basic\"" "Dashboard Tab" {
          tunnel: w223 -> [_ _ w239 _ _]
          tunnel: "/TestMode/Automatic/" ("Name Pattern") -> [_ _ w238 _ _]
          tunnel: T19 [{"Operation"=enum."Clear", "Color Box"=14013909}, {"Operation"=enum."Clear", "Color Box"=14013909}, {"Operation"=enum."Clear", "Color Box"=14013909}, {"Operation"=enum."Clear", "Color Box"=14013909}, {"Operation"=enum."Update", "Color Box"=14013909}, {"Operation"=enum."Update", "Color Box"=16777215}, {"Operation"=enum."Clear", "Color Box"=14013909}, {"Operation"=enum."Clear", "Color Box"=14013909}, {"Operation"=enum."Clear", "Color Box"=14013909}] -> [_ _ w231 _ w255]
          tunnel: w220 -> [_ _ w230 _ w254]
          tunnel: u32[] [15790320, 15790320, 15790320, 15790320, 16777215, 16777215, 15790320, 15790320, 15790320] -> [_ _ _ _ w260]
          tunnel: w218 -> [_ _ _ _ w248]
          tunnel: w215 -> [_ w225 _ _ _]
          frame "Custom", Default {
          }
          frame "Basic" {
            n120 = call <vilib>:"WPI_DashboardUpdateNames.vi"("Controls on Tab"=w225) -> ()  [unwired: 11 in]
          }
          frame "Test" {
            w237 = -2 ("Active Item:Row Number")
            n121 = Index Array(array=w231, index=w230) -> (element=w232:T22)
            n122 = Unbundle(w232) -> ("Operation"=w233:enum16{"Update", "Clear"}, "Color Box"=w234:u32)
            n123 = call <vilib>:"NT Read String.vi"("Name"="/TestMode/TestName") -> ("String"=w228:string)  [unwired: 9 in, 1 out]
            n124 = call <vilib>:"NT Read and Format Entries as Tree.vi"("Operation"=w233, "Name Pattern"=w238, "Tree Refnum"=w239) -> ()  [unwired: 7 in, 2 out]
            n125 = case shown="\"\"" w228 {
              tunnel: "/TestMode/TestProgress" ("Name") -> [w241 _]
              tunnel: "/TestMode/TestProgressText" ("Name") -> [w240 _]
              frame Default {
                n126 = call <vilib>:"NT Read Number.vi"("Name"=w241) -> ("Numeric"=w242:dbl)  [unwired: 9 in, 1 out]
                n127 = call <vilib>:"NT Read String.vi"("Name"=w240) -> ("String"=w243:string)  [unwired: 9 in, 1 out]
                n128 = Bundle("Numeric"=w242, "String"=w243) -> (→"Progress":cluster{"Numeric":dbl, "String":string})  [unwired: 1 in]
              }
              frame "" {
                n129 = property on="Progress" class="Clust (strict)"("Visible"=FALSE) -> ()  [unwired: 2 in, 2 out]
                n130 = local write "Test Name"(u16 0) -> ()
              }
            }
            n131 = property on="Test Tree" class="Tree (strict)"("Active Item Row Number"=w237, "ActiveColNum"=w237, "CellBG"=w234, "Active Item Row Number"=-1 ("Active Item:Row Number"), "CellBG"=u32 5789784 ("Color Box")) -> ()  [unwired: 2 in, 2 out]
          }
          frame "Variables" {
            n132 = control-ref of="Tree"() -> (w247:refnum<vi>)
            n133 = call <vilib>:"NT Read and Format Entries as Tree.vi"("Tree Refnum"=w247) -> ()  [unwired: 9 in, 2 out]
          }
          frame "Commands" {
            w256 = u32 5789784 ("Color Box")
            w257 = T23 {"Row"=-1, "Column"=-2} ("Active Cell:Active Cell")
            w259 = T23 {"Row"=-2, "Column"=-2} ("Active Cell:Active Cell")
            n134 = Index Array(array=w260, index=w254) -> (element=w258:u32)
            n135 = Index Array(array=w255, index=w254) -> (element=w253:T22)
            n136 = Unbundle(w253) -> ("Operation"=w252:enum16{"Update", "Clear"})  [unwired: 1 out]
            n137 = local read "Command Selection"() -> (w251:i32)
            n138 = property on="Command Selection" class="MCListbox (strict)"("ActiveCell"=w259, "CellBG"=w258, "ActiveCell"=w257, "CellBG"=w256) -> ()  [unwired: 2 in, 2 out]
            n139 = call <vilib>:"WPI_DashboardUpdate RPC Info.vi"("Operation"=w252) -> ("update"=w250:bool, "commands"=w249:string[][])  [unwired: 9 in]
            n140 = property on="Command Selection" class="MCListbox (strict)"("ItemNames"=w249) -> ()  [unwired: 2 in, 2 out]
            n141 = property on="Command Params" class="Tbl (strict)"("Active Cell"=w259, "Cell BG Color"=w258, "Active Cell"=w257, "Cell BG Color"=w256) -> ()  [unwired: 2 in, 2 out]
            n142 = call <vilib>:"WPI_DashboardUpdate Command Params.vi"("Update"=w250, "NewVal"=w251, "Commands"=w249, "Param Tbl"=w248) -> ()  [unwired: 7 in, 1 out]
          }
        }
        n143 = call <vilib>:"Connextion Info.vi"() -> ("Connected"=→"NT Connection":bool)  [unwired: 10 in, 1 out]
      }
      event "Test Tree": Value Change {
        # "Show appropriate\ncontrols"
        n144 = event-data() -> ("CtlRef"=w265:refnum<vi>, "NewVal"=w263:string)  [unwired: 1 in]
        n145 = call <vilib>:"WPI_UtilitiesGetTreeIOName.vi"("NewVal"=w263, "TreeControl in"=w265) -> ("I/O Name"=w266:string)  [unwired: 9 in]
        n146 = case shown="\"Camera\"" w266 {
          selector: w266 -> [_ w273 _ w295 w304 _]
          tunnel: w263 -> [_ _ w292 w294 _ w311]
          tunnel: cluster{string[]}[] [{["640x480", "320x240", "160x120"]}, {["Auto", "Fixed indoor", "Fixed outdoor 1", "Fixed outdoor 2", "Fixed fluorescent 1", "Fixed fluorescent 2", "Hold current"]}, {["Auto", "Flicker-free 50 Hz", "Flicker-free 60 Hz", "Hold current"]}, {["None", "Prioritize frame rate", "Prioritize image quality"]}, {["Monochrome", "Color"]}] -> [_ _ _ _ _ w310]
          frame Default {
            w268 = FALSE ("Visible")
            w267 = FALSE ("Visible")
            n147 = property on="Motor" class="Clust (strict)"("Visible"=w267) -> ()  [unwired: 2 in, 2 out]
            n148 = property on="Test Ring" class="Ring (strict)"("Visible"=w267) -> ()  [unwired: 2 in, 2 out]
            n149 = property on="Rev/Fwd" class="Clust (strict)"("Visible"=w268) -> ()  [unwired: 2 in, 2 out]
            n150 = property on="On/Off" class="Bool (strict)"("Visible"=w268) -> ()  [unwired: 2 in, 2 out]
            n151 = property on="Test Slider" class="Slide (strict)"("Visible"=w268) -> ()  [unwired: 2 in, 2 out]
          }
          frame "Analog Out", "Motor", "PWM" {
            w274 = FALSE ("Visible")
            n152 = case shown="\"Analog Out\"" w273 {
              tunnel: [1.0 ("Value") -1.0 ("Value") 0.0 ("Value")] -> w272
              tunnel: [255.0 ("Value") 1.0 ("Value") 5.0 ("Value")] -> w271
              tunnel: [128.0 ("Value") 0.0 ("Value") 0.0 ("Value")] -> w270
              tunnel: [64.0 ("Value") 0.5 ("Value") 1.0 ("Value")] -> w269
              frame "PWM" {
              }
              frame "Motor", Default {
              }
              frame "Analog Out" {
              }
            }
            n153 = property on="Motor" class="Clust (strict)"("Visible"=TRUE) -> ()  [unwired: 2 in, 2 out]
            n154 = property on="Value" class="Slide (strict)"("Value"=w270, "Scale.Minimum"=w272, "Scale.Maximum"=w271, "Scale.Increment"=w269) -> ()  [unwired: 2 in, 2 out]
            n155 = property on="On/Off" class="Bool (strict)"("Visible"=w274) -> ()  [unwired: 2 in, 2 out]
            n156 = property on="Test Slider" class="Slide (strict)"("Visible"=w274) -> ()  [unwired: 2 in, 2 out]
            n157 = property on="Test Ring" class="Ring (strict)"("Visible"=w274) -> ()  [unwired: 2 in, 2 out]
            n158 = property on="Rev/Fwd" class="Clust (strict)"("Visible"=w274) -> ()  [unwired: 2 in, 2 out]
          }
          frame "Servo" {
            w290 = FALSE ("Visible")
            n159 = call <vilib>:"NT Read Number.vi"("Name"=w292) -> ("Numeric"=w291:dbl)  [unwired: 9 in, 1 out]
            n160 = property on="Test Slider" class="Slide (strict)"("Visible"=TRUE, "Scale.Maximum"=170.0 ("Scale.Range:Maximum")) -> ()  [unwired: 2 in, 2 out]
            n161 = local write "Test Slider"(w291) -> ()
            n162 = property on="Motor" class="Clust (strict)"("Visible"=w290) -> ()  [unwired: 2 in, 2 out]
            n163 = property on="Rev/Fwd" class="Clust (strict)"("Visible"=w290) -> ()  [unwired: 2 in, 2 out]
            n164 = property on="On/Off" class="Bool (strict)"("Visible"=w290) -> ()  [unwired: 2 in, 2 out]
            n165 = property on="Test Ring" class="Ring (strict)"("Visible"=w290) -> ()  [unwired: 2 in, 2 out]
          }
          frame "Relay", "Solenoid" {
            w293 = FALSE ("Visible")
            n166 = property on="Motor" class="Clust (strict)"("Visible"=w293) -> ()  [unwired: 2 in, 2 out]
            n167 = property on="Test Slider" class="Slide (strict)"("Visible"=w293) -> ()  [unwired: 2 in, 2 out]
            n168 = Search and Replace String(input string=w294, search string="/Value  **", replace string="/Direction") -> (result string=w300:string)  [unwired: 5 in, 3 out]
            n169 = property on="Test Ring" class="Ring (strict)"("Visible"=w293) -> ()  [unwired: 2 in, 2 out]
            n170 = call <vilib>:"NT Read String.vi"("Name"=w300) -> ("String"=w298:string)  [unwired: 9 in, 1 out]
            n171 = Equal?(x="Both directions", y=w298) -> (x = y?=w296:bool)
            n172 = Not(x=w296) -> (.not. x?=w297:bool)
            n173 = property on="Rev/Fwd" class="Clust (strict)"("Visible"=w296) -> ()  [unwired: 2 in, 2 out]
            n174 = property on="On/Off" class="Bool (strict)"("Visible"=w297, "Caption.Text"=w295) -> ()  [unwired: 2 in, 2 out]
          }
          frame "Compressor", "Digital Out" {
            w303 = FALSE ("Visible")
            # "Get direction and finish"
            n175 = property on="Motor" class="Clust (strict)"("Visible"=w303) -> ()  [unwired: 2 in, 2 out]
            n176 = property on="Test Slider" class="Slide (strict)"("Visible"=w303) -> ()  [unwired: 2 in, 2 out]
            n177 = property on="Test Ring" class="Ring (strict)"("Visible"=w303) -> ()  [unwired: 2 in, 2 out]
            n178 = property on="On/Off" class="Bool (strict)"("Visible"=TRUE, "Caption.Text"=w304) -> ()  [unwired: 2 in, 2 out]
            n179 = property on="Rev/Fwd" class="Clust (strict)"("Visible"=FALSE) -> ()  [unwired: 2 in, 2 out]
          }
          frame "Camera" {
            n180 = call <vilib>:"Get Last Path Segment.vi"("String in"=w311) -> ("String out"=w312:string)  [unwired: 10 in]
            n181 = property on="On/Off" class="Bool (strict)"("Visible"=FALSE) -> ()  [unwired: 2 in, 2 out]
            n182 = property on="Motor" class="Clust (strict)"("Visible"=FALSE) -> ()  [unwired: 2 in, 2 out]
            n183 = property on="Rev/Fwd" class="Clust (strict)"("Visible"=FALSE) -> ()  [unwired: 2 in, 2 out]
            n184 = case shown="\"White Balance  **\"" w312 {
              tunnel: w311 -> [w318 w327 w336 w345 w354 _ w360]
              tunnel: w310 -> [w316 w324 w333 w342 w351 _ _]
              frame "Size  **" {
                n185 = Index Array(array=w316) -> (element=w315:cluster{string[]})  [unwired: 1 in]
                n186 = call <vilib>:"NT Read String.vi"("Name"=w318) -> ("String"=w317:string)  [unwired: 9 in, 1 out]
                n187 = Unbundle(w315) -> (w313:string[])
                n188 = Match First String(2:w313, 3:w317) -> (0:w314:i32)  [unwired: 1 out]
                n189 = property on="Test Ring" class="Ring (strict)"("Value"=w314, "Strings []"=w313) -> ()  [unwired: 2 in, 2 out]
                n190 = property on="Test Ring" class="Ring (strict)"("Visible"=TRUE) -> ()  [unwired: 2 in, 2 out]
                n191 = property on="Test Slider" class="Slide (strict)"("Visible"=FALSE) -> ()  [unwired: 2 in, 2 out]
              }
              frame "White Balance  **" {
                n192 = Index Array(array=w324, index=1) -> (element=w325:cluster{string[]})
                n193 = call <vilib>:"NT Read String.vi"("Name"=w327) -> ("String"=w326:string)  [unwired: 9 in, 1 out]
                n194 = Unbundle(w325) -> (w322:string[])
                n195 = Match First String(2:w322, 3:w326) -> (0:w321:i32)  [unwired: 1 out]
                n196 = property on="Test Ring" class="Ring (strict)"("Value"=w321, "Strings []"=w322) -> ()  [unwired: 2 in, 2 out]
                n197 = property on="Test Ring" class="Ring (strict)"("Visible"=TRUE) -> ()  [unwired: 2 in, 2 out]
                n198 = property on="Test Slider" class="Slide (strict)"("Visible"=FALSE) -> ()  [unwired: 2 in, 2 out]
              }
              frame "Exposure  **" {
                n199 = Index Array(array=w333, index=2) -> (element=w334:cluster{string[]})
                n200 = call <vilib>:"NT Read String.vi"("Name"=w336) -> ("String"=w335:string)  [unwired: 9 in, 1 out]
                n201 = Unbundle(w334) -> (w330:string[])
                n202 = Match First String(2:w330, 3:w335) -> (0:w331:i32)  [unwired: 1 out]
                n203 = property on="Test Ring" class="Ring (strict)"("Value"=w331, "Strings []"=w330) -> ()  [unwired: 2 in, 2 out]
                n204 = property on="Test Ring" class="Ring (strict)"("Visible"=TRUE) -> ()  [unwired: 2 in, 2 out]
                n205 = property on="Test Slider" class="Slide (strict)"("Visible"=FALSE) -> ()  [unwired: 2 in, 2 out]
              }
              frame "Exposure Priority  **" {
                n206 = Index Array(array=w342, index=3) -> (element=w343:cluster{string[]})
                n207 = call <vilib>:"NT Read String.vi"("Name"=w345) -> ("String"=w344:string)  [unwired: 9 in, 1 out]
                n208 = Unbundle(w343) -> (w339:string[])
                n209 = Match First String(2:w339, 3:w344) -> (0:w340:i32)  [unwired: 1 out]
                n210 = property on="Test Ring" class="Ring (strict)"("Value"=w340, "Strings []"=w339) -> ()  [unwired: 2 in, 2 out]
                n211 = property on="Test Ring" class="Ring (strict)"("Visible"=TRUE) -> ()  [unwired: 2 in, 2 out]
                n212 = property on="Test Slider" class="Slide (strict)"("Visible"=FALSE) -> ()  [unwired: 2 in, 2 out]
              }
              frame "Color Enable  **" {
                n213 = Index Array(array=w351, index=4) -> (element=w352:cluster{string[]})
                n214 = call <vilib>:"NT Read String.vi"("Name"=w354) -> ("String"=w353:string)  [unwired: 9 in, 1 out]
                n215 = Unbundle(w352) -> (w348:string[])
                n216 = Match First String(2:w348, 3:w353) -> (0:w349:i32)  [unwired: 1 out]
                n217 = property on="Test Ring" class="Ring (strict)"("Value"=w349, "Strings []"=w348) -> ()  [unwired: 2 in, 2 out]
                n218 = property on="Test Ring" class="Ring (strict)"("Visible"=TRUE) -> ()  [unwired: 2 in, 2 out]
                n219 = property on="Test Slider" class="Slide (strict)"("Visible"=FALSE) -> ()  [unwired: 2 in, 2 out]
              }
              frame Default {
                n220 = property on="Test Ring" class="Ring (strict)"("Visible"=FALSE) -> ()  [unwired: 2 in, 2 out]
                n221 = property on="Test Slider" class="Slide (strict)"("Visible"=FALSE) -> ()  [unwired: 2 in, 2 out]
              }
              frame "Brightness  **", "Color Level  **", "Compression  **", "FPS  **", "Sharpness  **" {
                n222 = call <vilib>:"NT Read Number.vi"("Name"=w360) -> ("Numeric"=w359:dbl)  [unwired: 9 in, 1 out]
                n223 = local write "Test Slider"(w359) -> ()
                n224 = property on="Test Slider" class="Slide (strict)"("Visible"=TRUE, "Scale.Maximum"=100.0 ("Scale.Range:Maximum")) -> ()  [unwired: 2 in, 2 out]
                n225 = property on="Test Ring" class="Ring (strict)"("Visible"=FALSE) -> ()  [unwired: 2 in, 2 out]
              }
            }
          }
        }
        n226 = property on="Progress" class="Clust (strict)"("Visible"=FALSE) -> ()  [unwired: 2 in, 2 out]
      }
      event "Test Name": Mouse Enter {
        # "Populate the ring with the list of tests"
        n227 = event-data() -> ()  [unwired: 1 in, 1 out]
        n228 = call <vilib>:"NT Read String Array.vi"("Name"="/TestMode/TestList") -> ("String Array"=w368:string[])  [unwired: 9 in, 1 out]
        n229 = Build Array (concatenate)("Select the test to run...", w368) -> (w367:string[])
        n230 = property on="Test Name" class="Ring (strict)"("Strings []"=w367) -> ()  [unwired: 2 in, 2 out]
      }
      event "Test Name": Value Change {
        w370 = FALSE ("Visible")
        # "Tell the robot the test name to run"
        n231 = event-data() -> ("NewVal"=w374:u16)  [unwired: 1 in]
        n232 = property on="Test Name" class="Ring (strict)"() -> ("Strings []"=w375:string[])  [unwired: 2 in, 2 out]
        n233 = local write "Progress"(T6 {"Test Progress"=0, "Test Progress Text"=""} ("Progress")) -> ()
        n234 = Index Array(array=w375, index=w374) -> (element=w373:string)
        n235 = call <vilib>:"NT Write String.vi"("String"=w373, "Name"="/TestMode/TestName") -> ()  [unwired: 9 in, 1 out]
        n236 = property on="Progress" class="Clust (strict)"("Visible"=TRUE) -> ()  [unwired: 2 in, 2 out]
        n237 = property on="Motor" class="Clust (strict)"("Visible"=w370) -> ()  [unwired: 2 in, 2 out]
        n238 = property on="Test Slider" class="Slide (strict)"("Visible"=w370) -> ()  [unwired: 2 in, 2 out]
        n239 = property on="On/Off" class="Bool (strict)"("Visible"=w370) -> ()  [unwired: 2 in, 2 out]
        n240 = property on="Rev/Fwd" class="Clust (strict)"("Visible"=w370) -> ()  [unwired: 2 in, 2 out]
        n241 = property on="Test Ring" class="Ring (strict)"("Visible"=w370) -> ()  [unwired: 2 in, 2 out]
      }
      event "Select Auto": Mouse Enter {
        # "Populate the combo box with the list of autonomous options"
        n242 = event-data() -> ()  [unwired: 1 in, 1 out]
        n243 = call <vilib>:"NT Read String Array.vi"("Name"="Auto List") -> ("String Array"=w377:string[])  [unwired: 9 in, 1 out]
        n244 = property on="Select Auto" class="CmbBox"("Strings[]"=w377) -> ()  [unwired: 2 in, 2 out]
      }
      event "Select Auto": Value Change {
        # "User modified the Auto Selection. Write to NT variable so robot knows."
        n245 = event-data() -> ("NewVal"=w380:string)  [unwired: 1 in]
        n246 = call <vilib>:"NT Write String.vi"("String"=w380, "Name"="Auto Selector") -> ()  [unwired: 9 in, 1 out]
      }
      event "Command Selection": Value Change {
        # "Get the params and show in table"
        n247 = event-data() -> ("NewVal"=w386:i32)  [unwired: 1 in]
        n248 = property on="Command Selection" class="MCListbox (strict)"() -> ("ItemNames"=w384:string[][])  [unwired: 2 in, 2 out]
        n249 = call <vilib>:"WPI_DashboardUpdate Command Params.vi"("NewVal"=w386, "Commands"=w384, "Param Tbl"=w385) -> ()  [unwired: 8 in, 1 out]
      }
      event "Execute Command": Value Change {
        # "Started one, Unique ID holds\nresponse"
        n250 = event-data() -> ()  [unwired: 1 in, 1 out]
        n251 = property on="Command Selection" class="MCListbox (strict)"() -> ("ItemNames"=w397:string[][])  [unwired: 2 in, 2 out]
        n252 = Index Array(array=w397, index (row)="Command Selection", index (col)=0) -> (element=w395:string)
        n253 = call <vilib>:"Invoke Commands.vi"("Command Params"="Command Params", "Function Name"=w395) -> ("Params"=w391:u8, "Started"=w390:bool)  [unwired: 7 in, 1 out]
        n254 = Array Subset(array="Command Params", length (row)=w391) -> (w392:string[][])  [unwired: 3 in]
        n255 = Select(t="Executing" ("Cmd Status"), s=w390, f="" ("Cmd Status")) -> (s? t:f=→"Cmd Status":string)
      }
      event "Command Selection": Double Click {
        n256 = event-data() -> ("Row"=w405:i32)  [unwired: 1 in]
        n257 = property on="Command Selection" class="MCListbox (strict)"() -> ("ItemNames"=w408:string[][])  [unwired: 2 in, 2 out]
        n258 = local read "Command Params"() -> (w404:string[][])
        n259 = Index Array(array=w408, index (row)=w405, index (col)=0) -> (element=w406:string)
        n260 = call <vilib>:"Invoke Commands.vi"("Command Params"=w404, "Function Name"=w406) -> ("Params"=w403:u8, "Started"=w398:bool)  [unwired: 7 in, 1 out]
        n261 = Array Subset(array=w404, length (row)=w403) -> (w402:string[][])  [unwired: 3 in]
        n262 = Select(t="Executing" ("Cmd Status"), s=w398, f="" ("Cmd Status")) -> (s? t:f=w399:string)
        n263 = local write "Cmd Status"(w399) -> ()
      }
      event "CheckList": Double Click {
        # "Shift clears all"
        # "Update symbols on the listbox"
        n264 = event-data() -> ("PlatMods.Shift"=w410:bool, "Row"=w412:i32)  [unwired: 1 in]
        n265 = case shown="True" w410 {
          tunnel: w412 -> [w416 _]
          tunnel: 1 -> [w415 _]
          frame False {
            n266 = property on="CheckList" class="LstBox (strict)"() -> ("Item Symbols"=w414:i32[])  [unwired: 2 in, 2 out]
            n267 = Replace Array Subset(array=w414, new element=w415, index=w416) -> (w413:i32[])
            n268 = property on="CheckList" class="LstBox (strict)"("Item Symbols"=w413) -> ()  [unwired: 2 in, 2 out]
          }
          frame True {
            w417 = 0 ("Top Row")
            n269 = property on="CheckList" class="LstBox (strict)"() -> ("Number of Rows"=w419:u32)  [unwired: 2 in, 2 out]
            n270 = Initialize Array(0, w419) -> (w418:i32[])
            n271 = property on="CheckList" class="LstBox (strict)"("Top Row"=w417, "Value"=w417, "Item Symbols"=w418) -> ()  [unwired: 2 in, 2 out]
          }
        }
      }
      event "CheckList": Key Down {
        # "Update symbols on the listbox\nLeft and right keys check and uncheck"
        n272 = event-data() -> ("VKey"=w423:T20)  [unwired: 1 in]
        n273 = case shown="\"Left\", \"Right\"" w423 {
          selector: w423 -> [w428 _]
          tunnel: eventvkey."Left" ("VKey") -> [w426 _]
          frame "Left", "Right" {
            n274 = Equal?(x=w426, y=w428) -> (x = y?=w427:bool)
            n275 = Select(t=0, s=w427, f=1) -> (s? t:f=w429:i32)
            n276 = property on="CheckList" class="LstBox (strict)"() -> ("Item Symbols"=w432:i32[])  [unwired: 2 in, 2 out]
            n277 = Replace Array Subset(array=w432, new element=w429, index="CheckList") -> (w431:i32[])
            n278 = property on="CheckList" class="LstBox (strict)"("Item Symbols"=w431) -> ()  [unwired: 2 in, 2 out]
          }
          frame Default {
          }
        }
      }
      event "Motor.Enable": Value Change {
        # "When the test mode otor enable helper is set, update that\ntree row item's value"
        n279 = event-data() -> ("NewVal"=w438:bool)  [unwired: 1 in]
        n280 = Unbundle("Motor") -> ("Value"=w437:dbl)  [unwired: 1 out]
        n281 = Select(t=w437, s=w438, f=0.0) -> (s? t:f=w435:dbl)
        n282 = call <vilib>:"NT Write Number.vi"("Numeric"=w435, "Name"=w434) -> ()  [unwired: 9 in, 1 out]
      }
      event "Test Slider": Value Change {
        # "When the test mode slider helper is set, update that\ntree row item's value"
        n283 = event-data() -> ("NewVal"=w441:dbl)  [unwired: 1 in]
        n284 = call <vilib>:"NT Write Number.vi"("Numeric"=w441, "Name"=w442) -> ()  [unwired: 9 in, 1 out]
      }
      event "On/Off": Value Change {
        # "When the test mode on/off helper value is set, update that\ntree row item's value"
        n285 = event-data() -> ("NewVal"=w446:bool)  [unwired: 1 in]
        n286 = Boolean To (0,1)(Boolean=w446) -> (0, 1=w445:i16)
        n287 = call <vilib>:"NT Write Number.vi"("Numeric"=w445, "Name"=w444) -> ()  [unwired: 9 in, 1 out]
      }
      event "Rev/Fwd": Value Change {
        # "When the test mode helper value for relays is set, update that\ntree row item's value"
        n288 = event-data() -> ("NewVal.Forward"=w454:bool, "NewVal.Reverse"=w453:bool)  [unwired: 1 in]
        n289 = Boolean To (0,1)(Boolean=w454) -> (0, 1=w450:i16)
        n290 = Boolean To (0,1)(Boolean=w453) -> (0, 1=w452:i16)
        n291 = Negate(x=w452) -> (-x=w451:i16)
        n292 = Add(x=w450, y=w451) -> (x+y=w449:i16)
        n293 = call <vilib>:"NT Write Number.vi"("Numeric"=w449, "Name"=w448) -> ()  [unwired: 9 in, 1 out]
      }
      event "Test Ring": Value Change {
        # "When a test mode helper value is selected from the ring,\nset the tree item's variable to the string value"
        n294 = event-data() -> ("NewVal"=w458:u16)  [unwired: 1 in]
        n295 = property on="Test Ring" class="Ring (strict)"() -> ("Strings []"=w459:string[])  [unwired: 2 in, 2 out]
        n296 = Index Array(array=w459, index=w458) -> (element=w457:string)
        n297 = call <vilib>:"NT Write String.vi"("String"=w457, "Name"=w456) -> ()  [unwired: 9 in, 1 out]
      }
      event "Rec Mode": Value Change {
        # "Update globals for recording mode and path to read log from.\nClear when logging and let NetworkTables set path for vision to\nuse."
        n298 = event-data() -> ("NewVal"=w470:enum32{"Stop", "Record", "Playback"})  [unwired: 1 in]
        n299 = global write "WPI_DashboardLogging Global.vi" "Logging Filename"(path "") -> ()
        n300 = global write "WPI_DashboardLogging Global.vi" "Recording"(w470) -> ()
        n301 = case shown="\"Playback\"" w470 {
          tunnel: w469 -> [_ w472 w481]
          tunnel: [_ _ w480] -> w467
          tunnel: [_ _ w479] -> _
          tunnel: w465 -> [_ _ w477]
          tunnel: cluster{i32, i32} {-250, 170} -> [_ _ w476]
          tunnel: [_ _ T21 {"Image Size"=TRUE, "Image Type"=TRUE, "Pixel Value"=TRUE, "ROI Information"=TRUE, "Zoom Factor"=FALSE} ("Image Information Shown:All Elements")] -> w463
          tunnel: [_ _ TRUE ("Zoom Factor")] -> w462
          tunnel: w461 -> [_ _ w473]
          frame Default {
          }
          frame "Stop", "Record" {
            # "Place Window too"
            n302 = invoke class="VI" method="FP.Close"(reference=w472) -> (reference out=w471:refnum<vi>)  [unwired: 2 in, 2 out]
            n303 = invoke class="VI" method="Abort VI"(reference=w471) -> ()  [unwired: 2 in, 3 out]
          }
          frame "Playback" {
            n304 = call "Open Playback Panel.vi"("Offset"=w476, "DB VI Ref"=w477, "Playback in"=w481) -> ("Playback out"=w478:refnum<vi>)  [unwired: 8 in]
            n305 = register-events(w478, w473) -> (reference out=w480:refnum<event-registration>, error out=w479:errorcluster)  [unwired: 2 in]
          }
        }
        n306 = property on="Camera Image" class="ImageControl"("Image Information Shown"=w463, "Image Information Visible"=w462) -> ()  [unwired: 2 in, 2 out]
        n307 = call <vilib>:"WPI_DashboardNT Log FieldName Cache.vi"("Operation"=enum16{"Lookup/Add", "Index", "Clear"}."Clear") -> ()  [unwired: 8 in, 3 out]
      }
      event Panel Close {
        w483 = enum32{"Stop", "Record", "Playback"}."Stop" ("Rec Mode")
        # "Playback window has been closed, abort"
        n308 = event-data() -> ()  [unwired: 1 in, 4 out]
        n309 = local write "Rec Mode"(w483) -> ()
        n310 = global write "WPI_DashboardLogging Global.vi" "Recording"(w483) -> ()
      }
      event Panel Close {
        # "Abort playback window and ourself"
        n311 = event-data() -> ()  [unwired: 1 in, 4 out]
        n312 = invoke class="VI" method="FP.Close"(reference=w487) -> (reference out=w486:refnum<vi>)  [unwired: 2 in, 2 out]
        n313 = invoke class="VI" method="Abort VI"(reference=w486) -> (error out=w485:errorcluster)  [unwired: 2 in, 2 out]
        n314 = invoke class="VI" method="Abort VI"(error in=w485) -> ()  [unwired: 2 in, 3 out]
      }
      event User Event {
        n315 = event-data() -> ("IDs"=w494:cluster{"RPC field ID":u16, "Unique ID":u16}, "String"=w493:string)  [unwired: 1 in]
        n316 = Bundle("IDs"=w494, "String"=w493) -> (w492:T8)  [unwired: 1 in]
        n317 = call <vilib>:"Retrieve RPC Response.vi"("RPC Response"=w492) -> ("Output"=w490:string[][])  [unwired: 10 in]
        n318 = Build Array (concatenate)(w488, w490) -> (w489:string[][])
        n319 = local write "Command Params"(w489) -> ()
        n320 = local write "Cmd Status"("" ("Cmd Status")) -> ()
      }
      event "Tree": Double Click {
        n321 = event-data() -> ("PlatMods"=w498:T24, "Tag"=w497:string)  [unwired: 1 in]
        n322 = Unbundle(w498) -> ("Shift"=w496:bool)  [unwired: 4 out]
        n323 = Not(x=w496) -> (.not. x?=w495:bool)
        n324 = call <vilib>:"NT Update Persistence.vi"("Persistence"=w495, "Name"=w497) -> ()  [unwired: 9 in, 1 out]
      }
    }
  }
  n325 = while {
    tunnel: w64 -> [w501]
    i -> [w504]
    stop <- FALSE stop-if-true
    n326 = Wait (ms)(milliseconds to wait=u32 100) -> ()  [unwired: 1 out]
    n327 = case shown="\"Playback\"" "Rec Mode" {
      tunnel: w504 -> [_ _ w519]
      tunnel: [u32 2829099 ("Base Color") u32 11141120 ("Target Color") w508] -> w500
      frame "Stop", Default {
        # "Reset the color, extra updates don't cost much"
      }
      frame "Record" {
      }
      frame "Playback" {
        # "Playback"
        n328 = Quotient & Remainder(x=w519, y=u32 50 ("milliseconds to wait")) -> (x-y*floor(x/y)=w515:u32)  [unwired: 1 out]
        n329 = Divide(x=w515, y=u32 50 ("milliseconds to wait")) -> (x/y=w512:dbl)
        n330 = Multiply(x=6.283185307179586, y=w512) -> (x*y=w517:dbl)
        n331 = Sine(x=w517) -> (sin(x)=w516:dbl)
        n332 = Absolute Value(x=w516) -> (abs(x)=w509:dbl)
        n333 = call "Interpolate RGB Color.vi"("Proportion"=w509, "Target Color"=u32 30976, "Base Color"=u32 2829099) -> ("Result Color"=w508:u32)  [unwired: 8 in]
      }
    }
    n334 = property class="Pane"(reference=w501, "PaneColor"=w500) -> ()  [unwired: 1 in, 2 out]
  }
  n335 = local write "Dashboard Tab"(T2."Drive" ("Dashboard Tab")) -> ()
  n336 = property on="On/Off" class="Bool (strict)"("Visible"=w33) -> ()  [unwired: 2 in, 2 out]
  n337 = property on="Motor" class="Clust (strict)"("Visible"=w33) -> ()  [unwired: 2 in, 2 out]
  n338 = property on="Progress" class="Clust (strict)"("Visible"=w33) -> ()  [unwired: 2 in, 2 out]
  n339 = property on="Test Ring" class="Ring (strict)"("Visible"=w33) -> ()  [unwired: 2 in, 2 out]
  n340 = property on="Rev/Fwd" class="Clust (strict)"("Visible"=w33) -> ()  [unwired: 2 in, 2 out]
  n341 = while {
    tunnel: u16 1741 ("timeout ms (25000)") -> [w521]
    stop <- FALSE stop-if-true
    n342 = TCP Create Listener(10:w521) -> (0:w520:errorcluster, 3:w522:refnum<k5>)  [unwired: 4 in, 1 out]
    n343 = case shown="No Error" w520 {
      selector: w520 -> [w524 _]
      tunnel: w522 -> [w525 _]
      frame No Error {
        n344 = while {
          tunnel: w525 -> [w528]
          tunnel: w524 -> [w527]
          stop <- FALSE stop-if-true
          n345 = TCP Wait On Listener(8:w527, 11:w528) -> (0:w529:errorcluster, 4:w530:refnum<k5>)  [unwired: 2 in, 3 out]
          n346 = local write "TCP"(w530) -> ()
          n347 = case shown="No Error" w529 {
            frame No Error {
            }
            frame Error {
              n348 = Wait (ms)(milliseconds to wait=u32 1000) -> ()  [unwired: 1 out]
            }
          }
        }
      }
      frame Error {
        n349 = Wait (ms)(milliseconds to wait=u32 1000) -> ()  [unwired: 1 out]
      }
    }
  }
  n350 = local write "Command Selection"(u16 0 ("milliseconds to wait")) -> ()
  n351 = local write "Command Params"(string[][] [] ("Command Params")) -> ()
  n352 = global write "WPI_DashboardLogging Global.vi" "Recording"(w58) -> ()
  n353 = local write "Rec Mode"(w58) -> ()
  n354 = call <vilib>:"NT Write String.vi"("String"="Select Auto", "Name"="Auto Selector") -> ()  [unwired: 9 in, 1 out]
